vi "Open.vi"(6 "clock_skew_threshold (1s)":dbl=1.0, 8 "error in":errorcluster, 9 "max_retries (3)":u32=3, 10 "TLS Config":T1, 11 "Connection Config":T2={"host"="localhost", "port"=9090, "username"="synnax", "password"="seldon"}) -> (0 "error out":errorcluster, 3 "Synnax Client out":refnum<class "Synnax Client.lvclass">)   [LabVIEW 2026, in "synnax_clib.lvlib" / "Synnax Client.lvclass"]
uses:
  Synnax Client.lvclass
  typedefs/connection_config.ctl
  typedefs/tls_config.ctl
  Synnax Client.lvclass/Synnax Client.ctl
  synnax_clib.lvlib
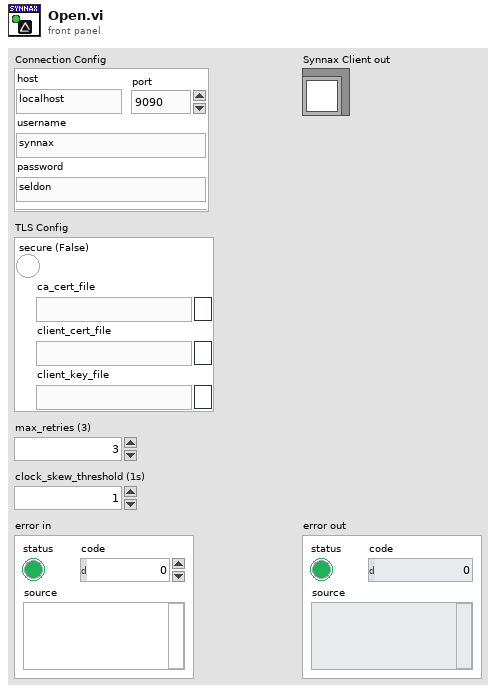
[diagram p1: front panel]
types:
  T1 = typedef "synnax_clib.lvlib/tls_config.ctl" = cluster{"secure (False)":bool, "ca_cert_file":path, "client_cert_file":path, "client_key_file":path}
  T2 = typedef "synnax_clib.lvlib/connection_config.ctl" = cluster{"host":string, "port":u16, "username":string, "password":string}
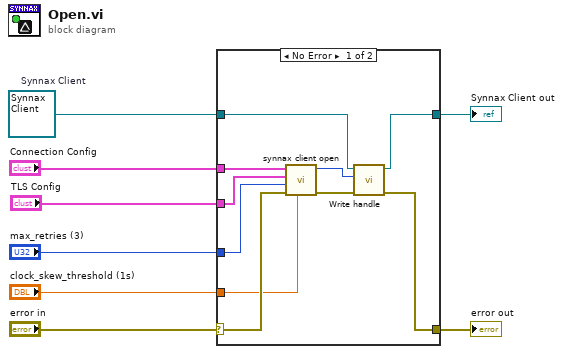
[diagram p0: block diagram]
diagram:
  w2 = refnum<class "Synnax Client.lvclass"> refnum  # Synnax Client
  n1 = case shown="No Error" "error in" {
    selector: "error in" -> [w17 w20]
    tunnel: "Connection Config" -> [w18 _]
    tunnel: "max_retries (3)" -> [w9 _]
    tunnel: "clock_skew_threshold (1s)" -> [w10 _]
    tunnel: [w15 w19] -> w3
    tunnel: [w13 w20] -> w4
    tunnel: w2 -> [w12 w19]
    tunnel: "TLS Config" -> [w11 _]
    frame No Error {
      n2 = call "synnax client open.vi"("clock_skew_threshold (1s)"=w10, "error in"=w17, "max_retries (3)"=w9, "TLS Config"=w11, "Connection Config"=w18) -> ("error out"=w14:errorcluster, "client handle out"=w16:u64)  [unwired: 5 in]
      n3 = call "Write handle.vi"("error in (no error)"=w14, "handle"=w16, "Synnax Client in"=w12) -> ("error out"=w13:errorcluster, "Synnax Client out"=w15:refnum<class "Synnax Client.lvclass">)  [unwired: 7 in]
    }
    frame Error {
    }
  }
  "error out" <- w4
  "Synnax Client out" <- w3
